vi "MTS_BuildWSTree.vi"(7 "Action":enum16{"Rebuild Tree", "Add to Tree"}(ring), 8 "error in":errorcluster, 10 "Files in Workspace":T1(array[cluster]), 11 "Tree Refnum":refnum<vi>) -> (0 "error out":errorcluster, 2 "numberOfFilesInWorkspace":i32, 3 "Tree Refnum (dup)":refnum<vi>)   [LabVIEW 2009]
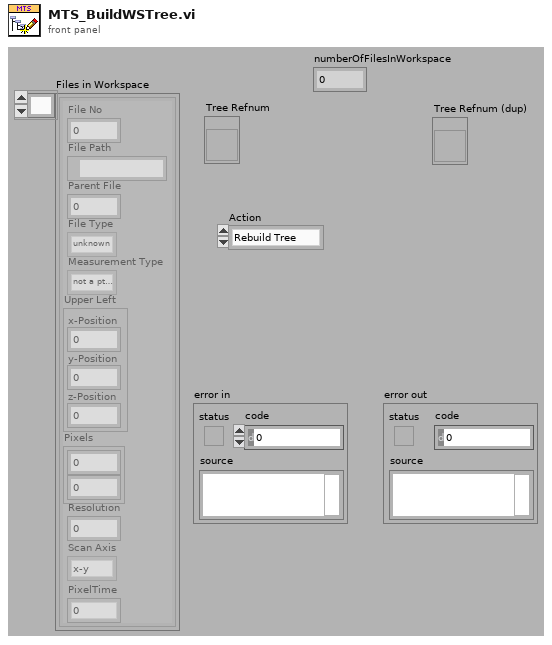
[diagram p1: front panel]
types:
  T1 = cluster{"File No":i32, "File Path":path, "Parent File":i32, "File Type":enum16{"unknown", "pt3 File", "png Image", "bmp Image"}, "Measurement Type":enum16{"not a pt3 File", "Image File", "Point Measurement", "Auto Point", "Line Scan", "Grid Scan"}, "Upper Left":cluster{"x-Position":dbl, "y-Position":dbl, "z-Position":dbl}, "Pixels":i32[], "Resolution":dbl, "Scan Axis":enum32{"x-y", "x-z", "y-x", "y-z", "z-x", "z-y"}, "PixelTime":dbl}[]
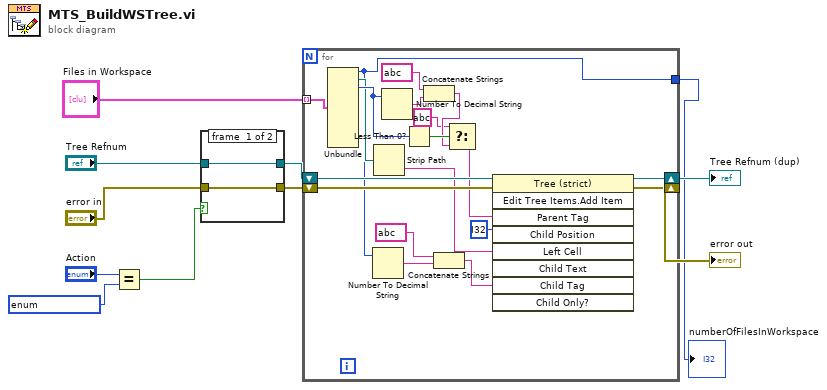
[diagram p0: block diagram]
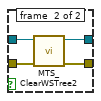
[diagram p2: hidden frame]
diagram:
  n1 = Equal?(x="Action", y=enum16{"Rebuild Tree", "Add to Tree"} ?) -> (x = y?=w2:bool)
  n2 = case shown="True" w2 {
    tunnel: "Tree Refnum" -> [w13 w17]
    tunnel: "error in" -> [w12 w16]
    tunnel: [w12 w15] -> w8
    tunnel: [w13 w14] -> w7
    frame #0 {
    }
    frame #1 {
      n3 = call "MTS_ClearWSTree2.vi"("error in"=w16, "Tree Refnum"=w17) -> ("error out"=w15:errorcluster, "Tree Refnum (dup)"=w14:refnum<vi>)  [unwired: 8 in]
    }
  }
  n4 = for {
    tunnel: "Files in Workspace" -> [w36] mode=indexing
    shift-right: [w31] -> w5
    shift-left: w8 -> [w33]
    shift-right: [w30] -> w6
    shift-left: w7 -> [w32]
    tunnel: [w18] -> w1
    n5 = Unbundle(w36) -> ("File No"=w18:i32, "File Path"=w22:path, "Parent File"=w28:i32)  [unwired: 7 out]
    n6 = Number To Decimal String(number=w18) -> (decimal integer string=w35:string)  [unwired: 1 in]
    n7 = Strip Path(path=w22) -> (name=w21:string)  [unwired: 1 out]
    n8 = Number To Decimal String(number=w28) -> (decimal integer string=w27:string)  [unwired: 1 in]
    n9 = Less Than 0?(x=w28) -> (x < 0?=w29:bool)
    n10 = Concatenate Strings(string ? ("decimal integer string"), w27) -> (w25:string)
    n11 = Concatenate Strings(string ? ("decimal integer string"), w35) -> (w20:string)
    n12 = Select(t=string ?, s=w29, f=w25) -> (s? t:f=w23:string)
    n13 = invoke on="Invoke Node" class="Tree (strict)" method="Edit Tree Items.Add Item"(reference=w32, error in=w33, "Parent Tag"=w23, "Child Position"=i32 ?, "Left Cell"=w21, "Child Tag"=w20) -> (reference out=w30:refnum<vi>, error out=w31:errorcluster)  [unwired: 3 in, 7 out]
  }
  "error out" <- w5
  "Tree Refnum (dup)" <- w6
  "numberOfFilesInWorkspace" <- w1
